vi "test Write File BIO.vi"(8 "error in (no error)":errorcluster, 11 "TestCase in":refnum<class "test BIO.lvclass">) -> (0 "error out":errorcluster, 3 "TestCase out":refnum<class "test BIO.lvclass">)   [LabVIEW 2013, in "test BIO.lvclass"]
uses:
  test BIO/test BIO.lvclass
  NI OpenSSL Socket/SSL_Lib/SSL-Lib/Library Paths.ctl
  <vilib>/addons/_JKI Toolkits/VI Tester/TestCase.llb/TestCase.lvclass
  NI OpenSSL Socket/SSL_Lib/SSL-Lib/SSL-Lib.lvclass
  NI OpenSSL Socket/SSL_Lib/BIO/BIO.lvclass
panel:
  out "return type":i32
  out "text":string
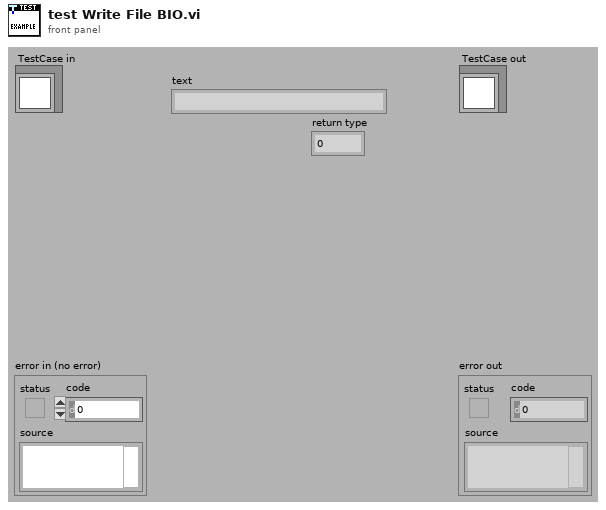
[diagram p1: front panel]
types:
  T1 = typedef "OpenSSL Socket.lvlib/SSL-Lib.lvclass/Library Paths.ctl" = cluster{"SSL Library Path":path, "Crypto Library Path":path}
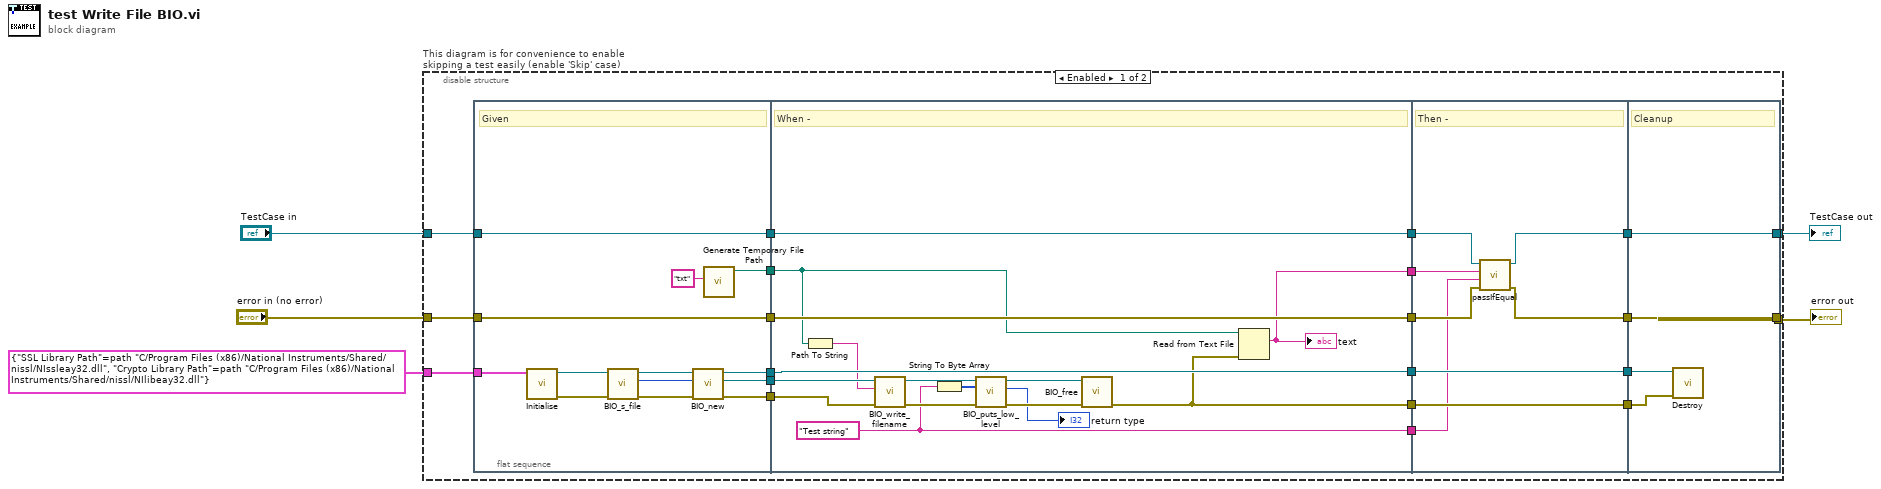
[diagram p0: block diagram]
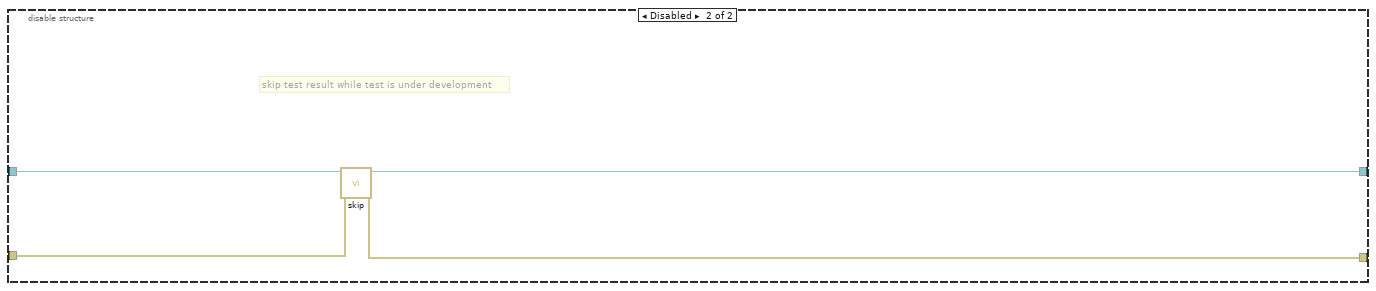
[diagram p2: hidden frame]
diagram:
  n1 = disable-structure "This diagram is for convenience to enable skipping a test easily (enable 'Skip' case)" shown="Enabled" {
    disable-tunnel: "TestCase in" -> [w19 w71]
    disable-tunnel: [w18 w69] -> w2
    disable-tunnel: [w17 w70] -> w4
    disable-tunnel: "error in (no error)" -> [w20 w68]
    disable-tunnel: T1 {"SSL Library Path"=path "C:/Program Files (x86)/National Instruments/Shared/nissl/NIssleay32.dll", "Crypto Library Path"=path "C:/Program Files (x86)/National Instruments/Shared/nissl/NIlibeay32.dll"} ("Library Paths") -> [w9 _]
    frame Enabled {
      n2 = flat-sequence {
        tunnel: w20 -> [w38]
        tunnel: w19 -> [w39]
        tunnel: [w39] -> w26
        tunnel: [w38] -> w25
        tunnel: [w32] -> w16
        tunnel: [w31] -> w15
        tunnel: [w30] -> w14
        tunnel: w9 -> [w29]
        tunnel: [w27] -> w8
        tunnel: [w55] -> w24
        tunnel: [w54] -> w23
        tunnel: w26 -> [w55]
        tunnel: w25 -> [w54]
        tunnel: w16 -> [w53]
        tunnel: w15 -> [w52]
        tunnel: w14 -> [w51]
        tunnel: [w51] -> w12
        tunnel: [w41] -> w10
        tunnel: w8 -> [w50]
        tunnel: [w48] -> w7
        tunnel: [w43] -> w6
        tunnel: [w62] -> w22
        tunnel: [w60] -> w21
        tunnel: w24 -> [w63]
        tunnel: w23 -> [w61]
        tunnel: [w59] -> w13
        tunnel: w12 -> [w59]
        tunnel: [w58] -> w11
        tunnel: w10 -> [w58]
        tunnel: w7 -> [w57]
        tunnel: w6 -> [w56]
        tunnel: [w66] -> w17
        tunnel: [w67] -> w18
        tunnel: w22 -> [w67]
        tunnel: w21 -> [w66]
        tunnel: w13 -> [w65]
        tunnel: w11 -> [w64]
        frame #0 {
          # "Given"
          n3 = call "Initialise.vi"("Library Paths"=w29) -> ("error out"=w34:errorcluster, "SSL-Lib out"=w35:refnum<class "SSL-Lib.lvclass">)  [unwired: 9 in]
          n4 = call "BIO_s_file.vi"("error in (no error)"=w34, "SSL-Lib in"=w35) -> ("error out"=w37:errorcluster, "*BIO_Method"=w33:u64, "SSL-Lib out"=w36:refnum<class "SSL-Lib.lvclass">)  [unwired: 7 in]
          n5 = call "BIO_new.vi"("error in (no error)"=w37, "*BIO_method"=w33, "SSL-Lib in"=w36) -> ("error out"=w31:errorcluster, "BIO out"=w32:refnum<class "BIO.lvclass">, "SSL-Lib out"=w30:refnum<class "SSL-Lib.lvclass">)  [unwired: 6 in]
          n6 = call <vilib>:"Generate Temporary File Path.vi"("Temporary File Extension (tmp)"="txt") -> ("Unique Temporary File Path"=w27:path)  [unwired: 9 in, 1 out]
        }
        frame #1 {
          w43 = "Test string" ("String to write")
          # "When -"
          n7 = Path To String(path=w50) -> (string=w49:string)
          n8 = call "BIO_write_filename.vi"("error in (no error)"=w52, "File path"=w49, "BIO in"=w53) -> ("error out"=w47:errorcluster, "BIO out"=w45:refnum<class "BIO.lvclass">)  [unwired: 7 in]
          n9 = String To Byte Array(string=w43) -> (unsigned byte array=w40:u8[])
          n10 = call "BIO_puts_low_level.vi"("error in (no error)"=w47, "Bytes to write"=w40, "BIO in"=w45) -> ("error out"=w46:errorcluster, "return type"=→"return type":i32, "BIO out"=w44:refnum<class "BIO.lvclass">)  [unwired: 6 in]
          n11 = call "BIO_free.vi"("error in (no error)"=w46, "BIO in"=w44) -> ("error out"=w41:errorcluster)  [unwired: 8 in, 1 out]
          n12 = Read from Text File(file (use dialog)=w50, error in=w41) -> (text=w48:string)  [unwired: 2 in, 3 out]
          "text" <- w48
        }
        frame #2 {
          # "Then -"
          n13 = call-dynamic "passIfEqual.vi"("error in (no error)"=w61, "y"=w56, "x"=w57, "TestCase in"=w63) -> ("error out"=w60:errorcluster, "TestCase out"=w62:refnum<class "test BIO.lvclass">)  [unwired: 6 in]
        }
        frame #3 {
          # "Cleanup"
          n14 = call "Destroy.vi"("error in (no error)"=w64, "SSL-Lib in"=w65) -> ()  [unwired: 9 in, 1 out]
        }
      }
    }
    frame Disabled {
      # "skip test result while test is under development"
      n15 = call <vilib>:"skip.vi"("error in (no error)"=w68, "TestCase in"=w71) -> ("error out"=w70:errorcluster, "TestCase out"=w69:refnum<class "test BIO.lvclass">)  [unwired: 8 in]
    }
  }
  "error out" <- w4
  "TestCase out" <- w2
